vi "CryoServer Read Buffered.vi"(8 "error in (no error)":errorcluster, 10 "timeout ms (5000)":i32=5000, 11 "connection ID":refnum<k5>) -> (0 "error out":errorcluster, 1 "messages":string[](array[string]), 2 "data out":string, 3 "connection ID out":refnum<k5>)   [LabVIEW 2024]
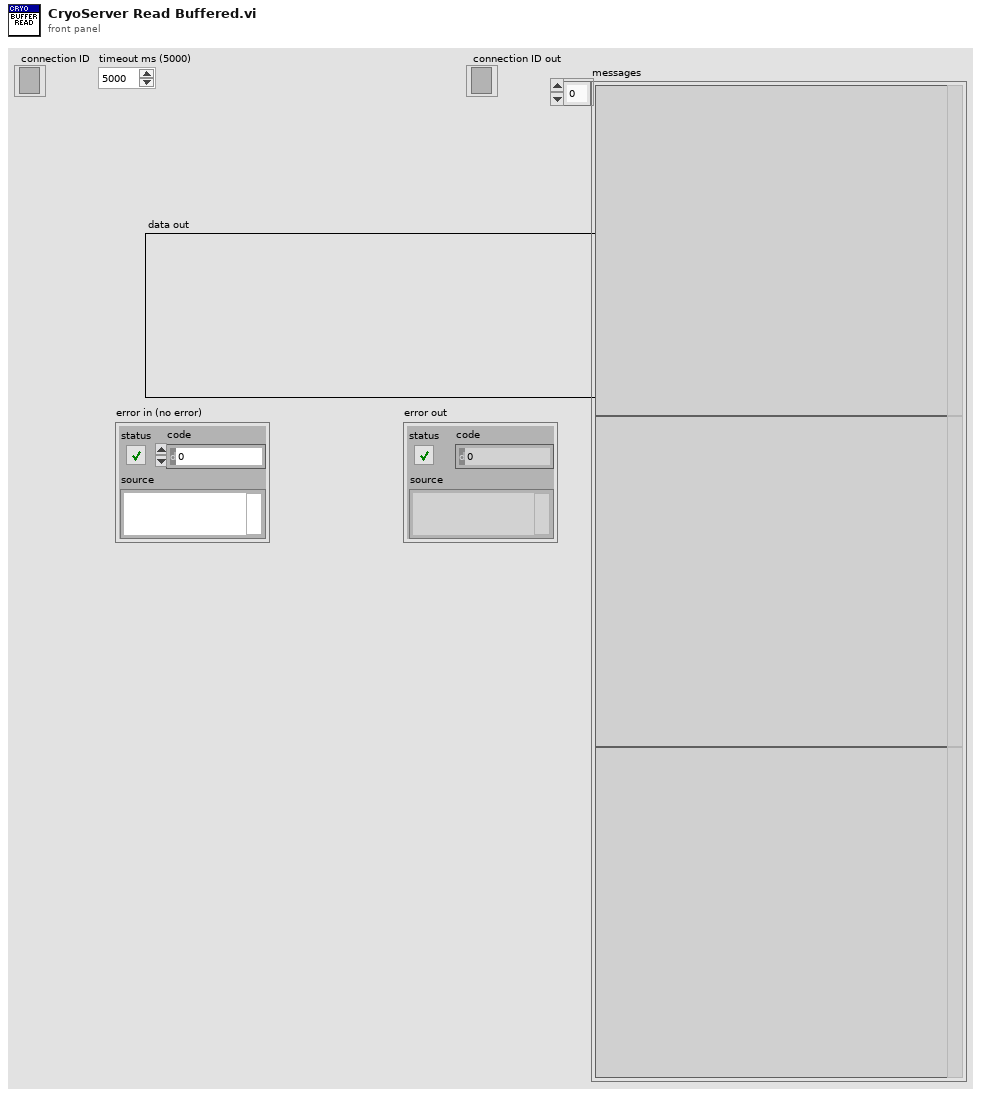
[diagram p1: front panel]
types:
  T1 = enum16{"Standard", "Buffered", "CRLF", "Immediate"}
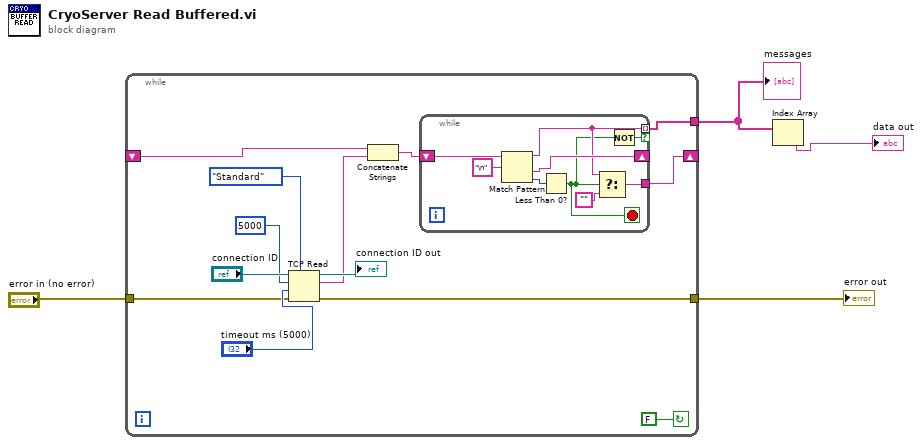
[diagram p0: block diagram]
diagram:
  n1 = while {
    tunnel: "error in (no error)" -> [w12]
    shift-right: [w5] -> _
    shift-left: _ -> [w6]
    tunnel: [w9] -> w2
    tunnel: [w8] -> w3
    stop <- FALSE continue-if-true
    n2 = TCP Read(connection ID="connection ID", bytes to read=5000, error in (no error)=w12, 7:T1."Standard" ("mode (standard)"), 9:"timeout ms (5000)") -> (connection ID out=→"connection ID out":refnum<k5>, data out=w11:string, error out=w8:errorcluster)
    n3 = Concatenate Strings(w6, w11) -> (w7:string)
    n4 = while {
      shift-right: [w23] -> _
      shift-left: w7 -> [w26]
      tunnel: [w22] -> w9 mode=indexing if=w18
      tunnel: [w20] -> w5
      stop <- w19 stop-if-true
      n5 = Match Pattern(string=w26, regular expression="\n") -> (before substring=w22:string, after substring=w23:string, offset past match=w24:i32)  [unwired: 1 in, 1 out]
      n6 = Less Than 0?(x=w24) -> (x < 0?=w19:bool)
      n7 = Select(t=w22, s=w19, f="") -> (s? t:f=w20:string)
      n8 = Not(x=w19) -> (.not. x?=w18:bool)
    }
  }
  "error out" <- w3
  "messages" <- w2
  n9 = Index Array(array=w2) -> (element=→"data out":string)  [unwired: 1 in]
